vi "Ageing test.vi"() -> ()   [LabVIEW 2014]
panel:
  out "Numeric":dbl
  out "CO Array":dbl[](array[numeric])
  out "Control type array":string[](array[string])
  in  "# of loops to run":i32
  out "total time":i32
  out "# of steps":i32
  out "# of repeats":i32
  out "loops":i32
  out "# of subcycles":i32
  out "# of cycles":i32
  out "Flow Rate":dbl
  out "Inlet Temp":dbl
  out "Bleed":dbl
  out "CO":dbl
  out "HC":dbl
  out "O2":dbl
  out "Inlet Lambda":dbl
  out "Bed Temp":dbl
  out "Time":dbl
  out "Contol type":string
  out "Finished?":bool
  out "Ageing Gas":i32
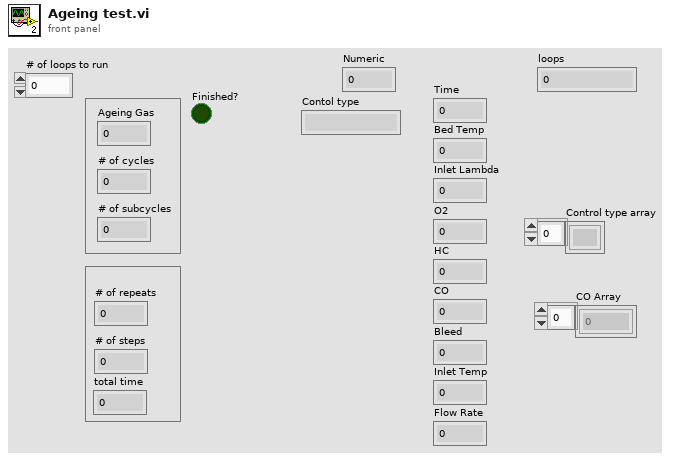
[diagram p1: front panel]
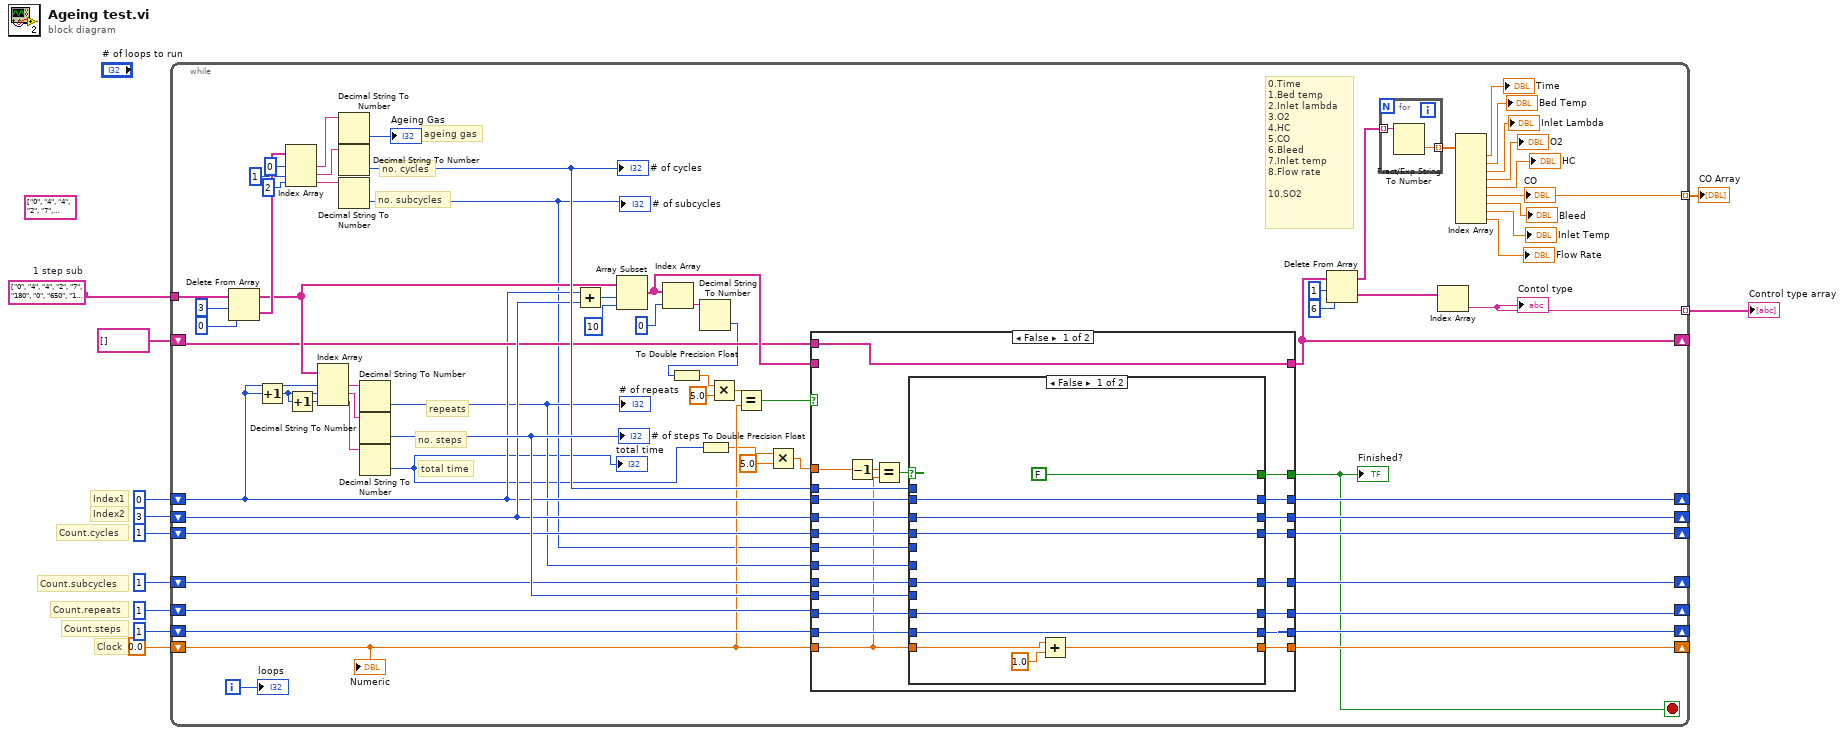
[diagram p0: block diagram]
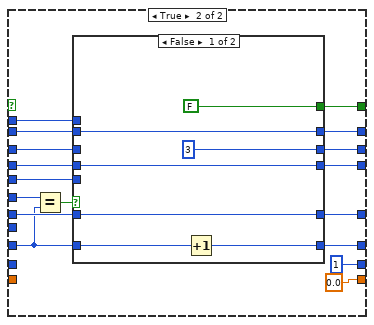
[diagram p2: hidden frame]
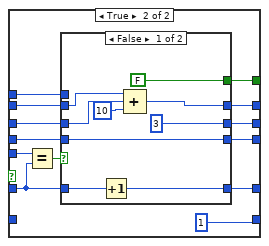
[diagram p3: hidden frame]
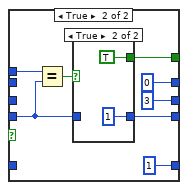
[diagram p4: hidden frame]
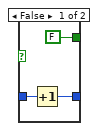
[diagram p5: hidden frame]
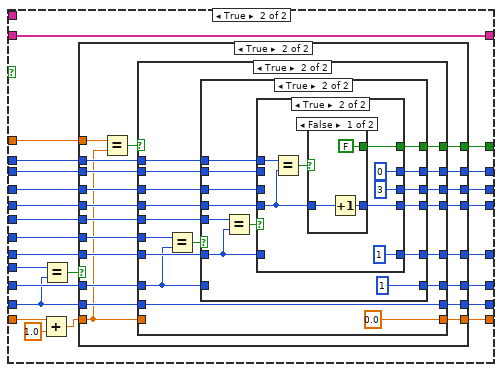
[diagram p6: hidden frame]
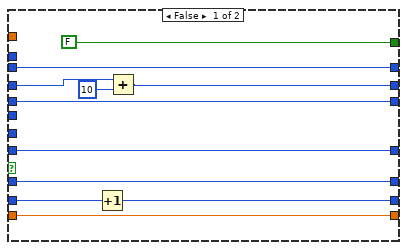
[diagram p7: hidden frame]
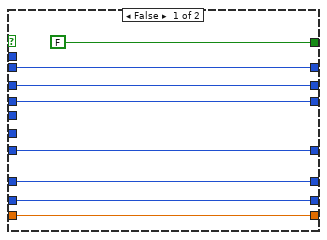
[diagram p8: hidden frame]
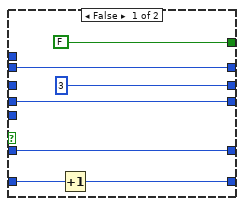
[diagram p9: hidden frame]
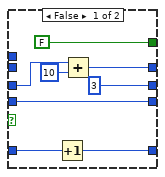
[diagram p10: hidden frame]
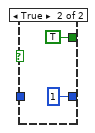
[diagram p11: hidden frame]
diagram:
  (unwired) string[] ["0", "4", "4", "2", "7", "180", "0", "650", "1", "0.5", " 0.111", "  1.00", "B", "0", "600", "15", "80", "650", "0.93", "0.03", " 0.334", "  3.00", "O", "0", "600", "15", "83", "650", "1", "0.5", " 0.111", "  1.00", "B", "0", "600", "15", "87", "650", "1", "0.5", " 0.111", "  1.00", "B", "0", "600", "15", "125", "650", "1.17", "2.9", " 0.004", "  0.04", "O", "0", "600", "15", "128", "650", "1", "0.5", " 0.111", "  1.00", "B", "0", "600", "15", "132", "650", "1", "0.5", " 0.111", "  1.00", "B", "0", "600", "15", "5", "2", "82", "0", "670", "1", "0.5", " 0.111", "  1.00", "B", "0", "600", "15", "80", "670", "0.93", "0.03", " 0.334", "  3.00", "O", "0", "600", "15", "9", "7", "180", "0", "650", "1", "0.5", " 0.111", "  1.00", "B", "0", "600", "15", "80", "650", "0.93", "0.03", " 0.334", "  3.00", "O", "0", "600", "15", "83", "650", "1", "0.5", " 0.111", "  1.00", "B", "0", "600", "15", "87", "650", "1", "0.5", " 0.111", "  1.00", "B", "0", "600", "15", "125", "650", "1.17", "2.9", " 0.004", "  0.04", "O", "0", "600", "15", "128", "650", "1", "0.5", " 0.111", "  1.00", "B", "0", "600", "15", "132", "650", "1", "0.5", " 0.111", "  1.00", "B", "0", "600", "15", "7", "2", "82", "0", "670", "1", "0.5", " 0.111", "  1.00", "B", "0", "600", "15", "80", "670", "0.93", "0.03", " 0.334", "  3.00", "O", "0", "600", "15"] ("appended array")
  w1 = string[] ["0", "4", "4", "2", "7", "180", "0", "650", "1", "0.5", " 0.111", "  1.00", "B", "0", "600", "15", "80", "650", "0.93", "0.03", " 0.334", "  3.00", "O", "0", "600", "15", "83", "650", "1", "0.5", " 0.111", "  1.00", "B", "0", "600", "15", "87", "650", "1", "0.5", " 0.111", "  1.00", "B", "0", "600", "15", "125", "650", "1.17", "2.9", " 0.004", "  0.04", "O", "0", "600", "15", "128", "650", "1", "0.5", " 0.111", "  1.00", "B", "0", "600", "15", "132", "650", "1", "0.5", " 0.111", "  1.00", "B", "0", "600", "15", "5", "1", "80", "0", "670", "1", "0.5", " 0.111", "  1.00", "B", "0", "600", "15", "9", "7", "180", "0", "650", "1", "0.5", " 0.111", "  1.00", "B", "0", "600", "15", "80", "650", "0.93", "0.03", " 0.334", "  3.00", "O", "0", "600", "15", "83", "650", "1", "0.5", " 0.111", "  1.00", "B", "0", "600", "15", "87", "650", "1", "0.5", " 0.111", "  1.00", "B", "0", "600", "15", "125", "650", "1.17", "2.9", " 0.004", "  0.04", "O", "0", "600", "15", "128", "650", "1", "0.5", " 0.111", "  1.00", "B", "0", "600", "15", "132", "650", "1", "0.5", " 0.111", "  1.00", "B", "0", "600", "15", "7", "1", "80", "0", "670", "1", "0.5", " 0.111", "  1.00", "B", "0", "600", "15"]  # 1 step sub
  # "Index2"
  # "Index1"
  # "Clock"
  # "Count.steps"
  # "Count.repeats"
  # "Count.subcycles"
  # "Count.cycles"
  n1 = while {
    shift-right: [w27] -> _
    shift-left: string[] [] ("Ageing Variables") -> [w51]
    shift-right: [w49] -> _
    shift-left: 0.0 -> [w22]
    shift-right: [w48] -> _
    shift-left: 1 -> [w56]
    shift-right: [w47] -> _
    shift-left: 1 -> [w55]
    shift-right: [w46] -> _
    shift-left: 1 -> [w54]
    shift-right: [w43] -> _
    shift-left: 0 -> [w24]
    shift-right: [w44] -> _
    shift-left: 3 -> [w52]
    shift-right: [w45] -> _
    shift-left: 1 -> [w53]
    tunnel: w1 -> [w28]
    tunnel: [w26] -> w3 mode=indexing
    tunnel: [w25] -> w2 mode=indexing
    i -> [w29]
    stop <- w20 stop-if-true
    # "total time"
    # "0.Time\n1.Bed temp\n2.Inlet lambda\n3.O2\n4.HC\n5.CO\n6.Bleed\n7.Inlet temp\n8.Flow rate\n\n10.SO2"
    # "ageing gas"
    # "repeats"
    # "no. steps"
    # "no. subcycles"
    # "no. cycles"
    n2 = Delete From Array(array=w28, length=3, index=0) -> (deleted portion=w77:string[], array with subset deleted=w60:string[])
    n3 = Increment(x=w24) -> (x+1=w70:i32)
    n4 = Index Array(array=w77, index #1=0 ("index"), index #2=1 ("index"), index #3=2 ("index")) -> (element #1=w76:string, element #2=w74:string, element #3=w75:string)
    n5 = Increment(x=w70) -> (x+1=w69:i32)
    n6 = Index Array(array=w60, index #1=w24, index #2=w70, index #3=w69) -> (element #1=w62:string, element #2=w63:string, element #3=w68:string)
    n7 = Decimal String To Number(string=w76) -> (number=→"Ageing Gas":i32)  [unwired: 2 in, 1 out]
    n8 = Decimal String To Number(string=w74) -> (number=w61:i32)  [unwired: 2 in, 1 out]
    "# of cycles" <- w61
    n9 = Decimal String To Number(string=w75) -> (number=w21:i32)  [unwired: 2 in, 1 out]
    "# of subcycles" <- w21
    n10 = Decimal String To Number(string=w62) -> (number=w23:i32)  [unwired: 2 in, 1 out]
    "# of repeats" <- w23
    n11 = Decimal String To Number(string=w63) -> (number=w71:i32)  [unwired: 2 in, 1 out]
    "# of steps" <- w71
    n12 = Decimal String To Number(string=w68) -> (number=w18:i32)  [unwired: 2 in, 1 out]
    "total time" <- w18
    n13 = Add(x=w24, y=w52) -> (x+y=w67:i32)
    n14 = Array Subset(array=w60, index=w67, length=10) -> (w73:string[])
    n15 = Index Array(array=w73, index=0) -> (element=w65:string)
    n16 = Decimal String To Number(string=w65) -> (number=w19:i32)  [unwired: 2 in, 1 out]
    n17 = To Double Precision Float(number=w19) -> (double precision float=w12:dbl)
    n18 = To Double Precision Float(number=w18) -> (double precision float=w17:dbl)
    n19 = Multiply(x=w12, y=5.0) -> (x*y=w13:dbl)
    n20 = Equal?(x=w13, y=w22) -> (x = y?=w72:bool)
    n21 = Multiply(x=w17, y=5.0) -> (x*y=w16:dbl)
    n22 = case shown="False" w72 {
      tunnel: w52 -> [w94 w197]
      tunnel: [w101 w196] -> w44
      tunnel: w22 -> [w85 w176]
      tunnel: [w96 w182] -> w49
      tunnel: w54 -> [w90 w191]
      tunnel: w56 -> [w88 w177]
      tunnel: [w87 w181] -> w48
      tunnel: w71 -> [w86 w194]
      tunnel: w24 -> [w89 w183]
      tunnel: w55 -> [w97 w178]
      tunnel: [w98 w185] -> w47
      tunnel: w23 -> [w91 w192]
      tunnel: [w99 w186] -> w46
      tunnel: w21 -> [w92 w190]
      tunnel: w53 -> [w93 w189]
      tunnel: w61 -> [w95 w188]
      tunnel: [w100 w187] -> w45
      tunnel: [w102 w184] -> w43
      tunnel: [w104 w195] -> w20
      tunnel: w16 -> [w82 w179]
      tunnel: [w84 w180] -> w27
      tunnel: w73 -> [_ w180]
      tunnel: w51 -> [w84 _]
      frame False {
        n23 = Decrement(x=w82) -> (x-1=w83:dbl)
        n24 = Equal?(x=w83, y=w85) -> (x = y?=w103:bool)
        n25 = case shown="False" w103 {
          tunnel: w97 -> [w109 w118]
          tunnel: w91 -> [_ w131]
          tunnel: w90 -> [w108 w129]
          tunnel: w92 -> [_ w128]
          tunnel: w93 -> [w111 w127]
          tunnel: w95 -> [_ w126]
          tunnel: [FALSE w125] -> w104
          tunnel: [w111 w121] -> w100
          tunnel: [w108 w119] -> w99
          tunnel: [w109 w117] -> w98
          tunnel: [w113 w124] -> w102
          tunnel: w94 -> [w112 w123]
          tunnel: [w112 w122] -> w101
          tunnel: w89 -> [w113 w120]
          tunnel: [w107 0.0] -> w96
          tunnel: w85 -> [w106 _]
          tunnel: w88 -> [w110 _]
          tunnel: [w110 1] -> w87
          tunnel: w86 -> [_ _]
          frame False {
            n26 = Add(x=w106, y=1.0) -> (x+y=w107:dbl)
          }
          frame True {
            n27 = Equal?(x=w131, y=w118) -> (x = y?=w130:bool)
            n28 = case shown="False" w130 {
              tunnel: w129 -> [w133 w141]
              tunnel: w128 -> [_ w151]
              tunnel: w127 -> [w134 w149]
              tunnel: w126 -> [_ w148]
              tunnel: [FALSE w147] -> w125
              tunnel: [w137 w146] -> w124
              tunnel: w123 -> [_ w145]
              tunnel: [3 w144] -> w122
              tunnel: [w134 w143] -> w121
              tunnel: w120 -> [w137 w142]
              tunnel: [w133 w140] -> w119
              tunnel: w118 -> [w136 _]
              tunnel: [w135 1] -> w117
              frame False {
                n29 = Increment(x=w136) -> (x+1=w135:i32)
              }
              frame True {
                n30 = Equal?(x=w151, y=w141) -> (x = y?=w150:bool)
                n31 = case shown="False" w150 {
                  tunnel: w149 -> [w155 w164]
                  tunnel: w148 -> [_ w168]
                  tunnel: [FALSE w166] -> w147
                  tunnel: [w160 0] -> w146
                  tunnel: w145 -> [w154 _]
                  tunnel: [3 ("y") 3] -> w144
                  tunnel: [w155 w165] -> w143
                  tunnel: w142 -> [w152 _]
                  tunnel: w141 -> [w157 _]
                  tunnel: [w156 1] -> w140
                  frame False {
                    n32 = Increment(x=w157) -> (x+1=w156:i32)
                    n33 = Compound Arithmetic op=ADD(w152, w154, 10 ("y")) -> (w160:i32)
                  }
                  frame True {
                    n34 = Equal?(x=w168, y=w164) -> (x = y?=w167:bool)
                    n35 = case shown="True" w167 {
                      tunnel: [FALSE TRUE] -> w166
                      tunnel: [w169 1] -> w165
                      tunnel: w164 -> [w170 _]
                      frame False {
                        n36 = Increment(x=w170) -> (x+1=w169:i32)
                      }
                      frame True {
                      }
                    }
                  }
                }
              }
            }
          }
        }
      }
      frame True {
        n37 = Add(x=w176, y=1.0) -> (x+y=w175:dbl)
        n38 = Equal?(x=w194, y=w177) -> (x = y?=w193:bool)
        n39 = case shown="True" w193 {
          tunnel: w197 -> [w200 w215]
          tunnel: [w201 w214] -> w196
          tunnel: [FALSE w220] -> w195
          tunnel: w179 -> [_ w228]
          tunnel: w178 -> [w203 w226]
          tunnel: w192 -> [_ w225]
          tunnel: w191 -> [w204 w224]
          tunnel: w190 -> [_ w223]
          tunnel: w189 -> [w205 w222]
          tunnel: w188 -> [_ w221]
          tunnel: w175 -> [w207 w209]
          tunnel: [w205 w219] -> w187
          tunnel: [w204 w218] -> w186
          tunnel: [w203 w217] -> w185
          tunnel: [w206 w216] -> w184
          tunnel: w183 -> [w206 w213]
          tunnel: [w207 w212] -> w182
          tunnel: w177 -> [w199 w210]
          tunnel: [w198 w211] -> w181
          frame False {
            n40 = Increment(x=w199) -> (x+1=w198:i32)
            n41 = Add(x=w200, y=10) -> (x+y=w201:i32)
          }
          frame True {
            n42 = Equal?(x=w228, y=w209) -> (x = y?=w227:bool)
            n43 = case shown="True" w227 {
              tunnel: w226 -> [w234 w240]
              tunnel: w225 -> [_ w253]
              tunnel: w224 -> [w235 w251]
              tunnel: w223 -> [_ w250]
              tunnel: w222 -> [w236 w249]
              tunnel: w221 -> [_ w248]
              tunnel: [FALSE w247] -> w220
              tunnel: [w236 w243] -> w219
              tunnel: [w235 w241] -> w218
              tunnel: [w234 w239] -> w217
              tunnel: [w231 w246] -> w216
              tunnel: w215 -> [w230 w245]
              tunnel: [w230 w244] -> w214
              tunnel: w213 -> [w231 w242]
              tunnel: [w232 0.0] -> w212
              tunnel: w209 -> [w232 _]
              tunnel: [w229 w237] -> w211
              tunnel: w210 -> [w229 w237]
              frame False {
              }
              frame True {
                n44 = Equal?(x=w253, y=w240) -> (x = y?=w252:bool)
                n45 = case shown="True" w252 {
                  tunnel: w251 -> [w256 w263]
                  tunnel: w250 -> [_ w273]
                  tunnel: w249 -> [w257 w271]
                  tunnel: w248 -> [_ w270]
                  tunnel: [FALSE w269] -> w247
                  tunnel: [w254 w268] -> w246
                  tunnel: w245 -> [_ w267]
                  tunnel: [3 ("y") w266] -> w244
                  tunnel: [w257 w265] -> w243
                  tunnel: w242 -> [w254 w264]
                  tunnel: [w256 w262] -> w241
                  tunnel: w240 -> [w259 _]
                  tunnel: [w258 1] -> w239
                  frame False {
                    n46 = Increment(x=w259) -> (x+1=w258:i32)
                  }
                  frame True {
                    n47 = Equal?(x=w273, y=w263) -> (x = y?=w272:bool)
                    n48 = case shown="True" w272 {
                      tunnel: w271 -> [w275 w285]
                      tunnel: w270 -> [_ w289]
                      tunnel: [FALSE w287] -> w269
                      tunnel: [w281 0] -> w268
                      tunnel: w267 -> [w280 _]
                      tunnel: [3 ("y") 3] -> w266
                      tunnel: [w275 w286] -> w265
                      tunnel: w264 -> [_ _]
                      tunnel: w263 -> [w277 _]
                      tunnel: [w276 1] -> w262
                      frame False {
                        n49 = Increment(x=w277) -> (x+1=w276:i32)
                        n50 = Add(x=w280, y=10) -> (x+y=w281:i32)
                      }
                      frame True {
                        n51 = Equal?(x=w289, y=w285) -> (x = y?=w288:bool)
                        n52 = case shown="False" w288 {
                          tunnel: [FALSE TRUE] -> w287
                          tunnel: [w290 1] -> w286
                          tunnel: w285 -> [w291 _]
                          frame False {
                            n53 = Increment(x=w291) -> (x+1=w290:i32)
                          }
                          frame True {
                          }
                        }
                      }
                    }
                  }
                }
              }
            }
          }
        }
      }
    }
    "Finished?" <- w20
    n54 = Delete From Array(array=w27, length=1, index=6) -> (deleted portion=w38:string[], array with subset deleted=w40:string[])
    n55 = for {
      tunnel: w40 -> [w81] mode=indexing
      tunnel: [w80] -> w39 mode=indexing
      n56 = Fract/Exp String To Number(string=w81) -> (number=w80:dbl)  [unwired: 3 in, 1 out]
    }
    n57 = Index Array(array=w38) -> (element=w26:string)  [unwired: 1 in]
    "Contol type" <- w26
    n58 = Index Array(array=w39) -> (element #1=→"Time":dbl, element #2=→"Bed Temp":dbl, element #3=→"Inlet Lambda":dbl, element #4=→"O2":dbl, element #5=→"HC":dbl, element #6=w25:dbl, element #7=→"Bleed":dbl, element #8=→"Inlet Temp":dbl, element #9=→"Flow Rate":dbl)  [unwired: 9 in]
    "CO" <- w25
    "loops" <- w29
    "Numeric" <- w22
  }
  "Control type array" <- w3
  "CO Array" <- w2
